vi "14-type_window.vi"(3 "this":i32, 4 "window in":i32, 5 "button":i32, 6 "settings in":T1={"Auto1"=TRUE, "Auto2"=TRUE, "Rel1"=TRUE, "Rel2"=TRUE, "Filt1"=TRUE, "Filt2"=TRUE, "Rate"=enum."Slow", "Range1"=enum."10mV", "Range2"=enum."100mV", "Filt3"=TRUE, "Filt4"=TRUE, "Rel temp 1"=TRUE, "Analog1"=FALSE, "Analog2"=FALSE, "Analog temp 1"=FALSE, "Digital1"=TRUE, "Digital2"=TRUE, "Digital temp 1 "=TRUE, "Window1"=enum."0,01%", "Window2"=enum."0,01%", "Window temp 1"=enum."0,01%", "RDGS1"="010", "RDGS2"="010", "RDGS temp 1"="010", "Type_type1"=TRUE, "Type_type2"=TRUE, "Type_type temp 1"=TRUE, "LSync"=FALSE, "Unit"=enum."C", "Sens"=TRUE, "Type tcoupl"=enum."J", "Junc"=TRUE, "prevState"=0, "Rel temp 2"=TRUE, "Analog temp 2"=FALSE, "Digital temp 2"=TRUE, "Type_type temp 2"=TRUE, "RDGS temp 2"="010", "Window temp 2"=enum."0,01%", "addres"=0}) -> (0 "next state":i32, 1 "window out":i32, 2 "settings out":T1)   [LabVIEW 2017]
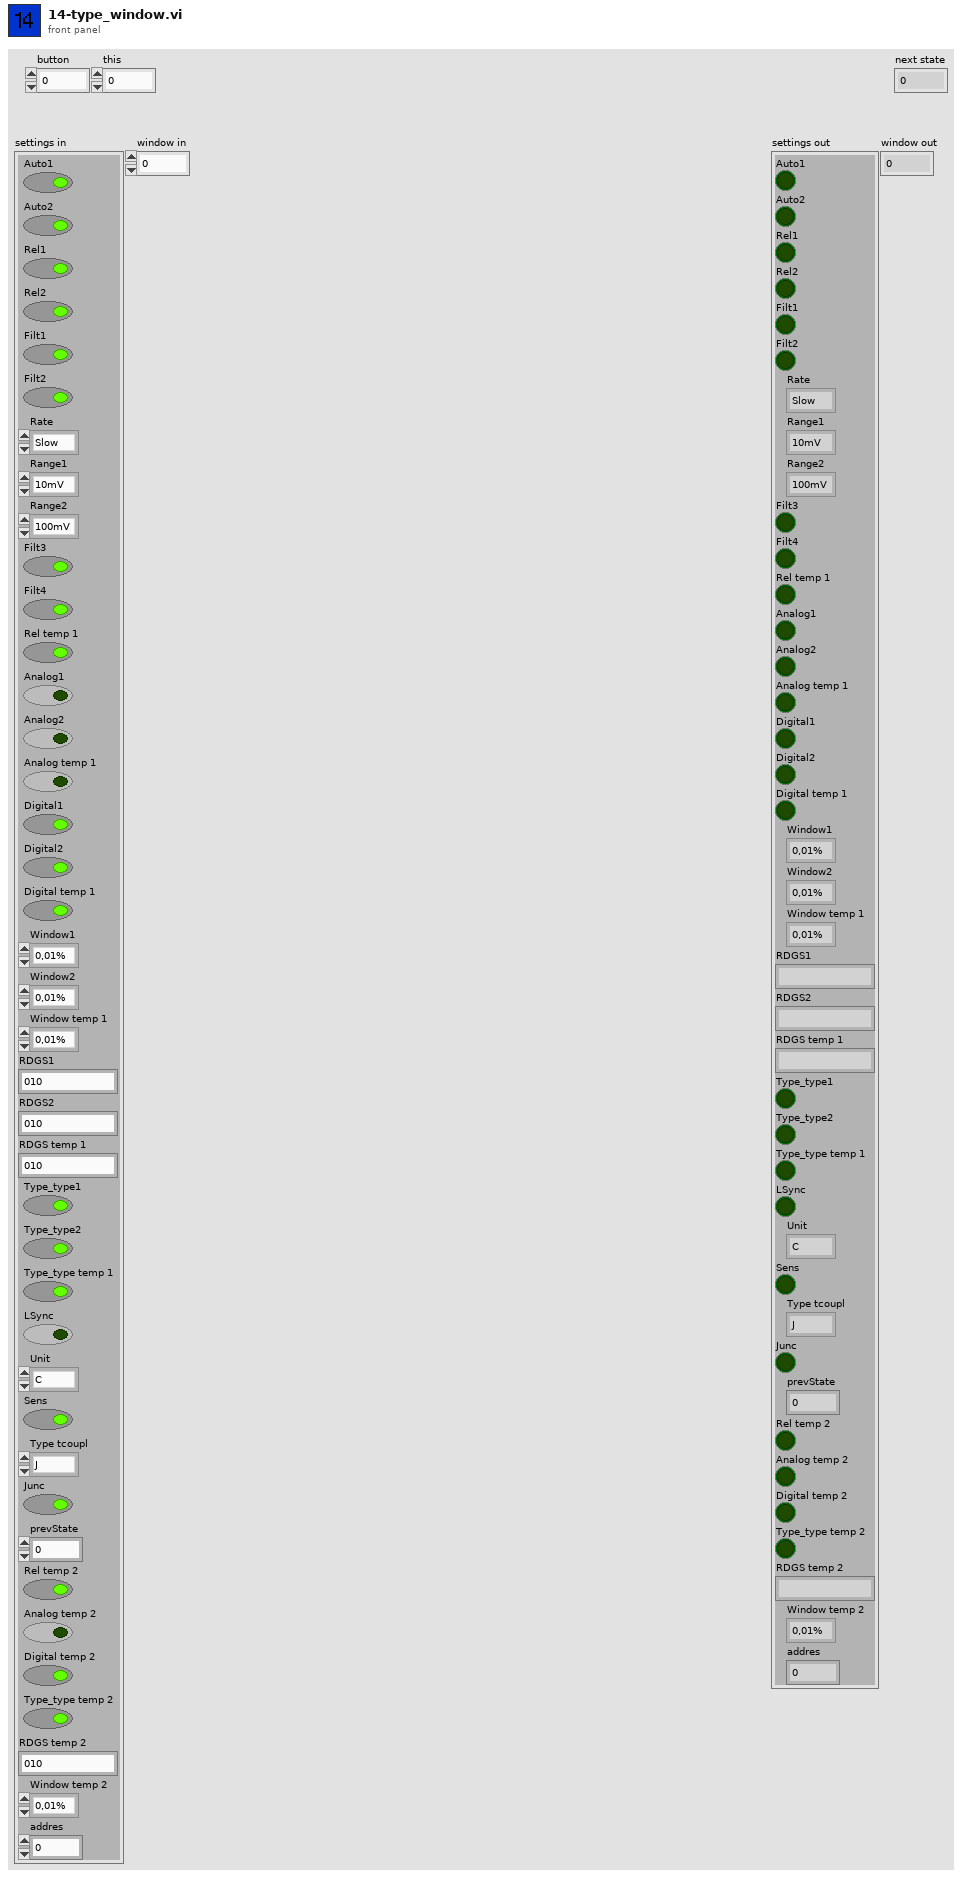
[diagram p1: front panel]
types:
  T1 = cluster{"Auto1":bool, "Auto2":bool, "Rel1":bool, "Rel2":bool, "Filt1":bool, "Filt2":bool, "Rate":enum16{"Slow", "Med", "Fast"}, "Range1":enum16{"10mV", "100mV", "1V", "10V", "100V"}, "Range2":enum16{"100mV", "1V", "10V"}, "Filt3":bool, "Filt4":bool, "Rel temp 1":bool, "Analog1":bool, "Analog2":bool, "Analog temp 1":bool, "Digital1":bool, "Digital2":bool, "Digital temp 1 ":bool, "Window1":enum16{"0,01%", "0,1%", "1%", "10%", "None"}, "Window2":enum16{"0,01%", "0,1%", "1%", "10%", "None"}, "Window temp 1":enum16{"0,01%", "0,1%", "1%", "10%", "None"}, "RDGS1":string, "RDGS2":string, "RDGS temp 1":string, "Type_type1":bool, "Type_type2":bool, "Type_type temp 1":bool, "LSync":bool, "Unit":enum16{"C", "K", "F"}, "Sens":bool, "Type tcoupl":enum16{"J", "K", "T", "E", "R", "S", "B", "N"}, "Junc":bool, "prevState":i32, "Rel temp 2":bool, "Analog temp 2":bool, "Digital temp 2":bool, "Type_type temp 2":bool, "RDGS temp 2":string, "Window temp 2":enum16{"0,01%", "0,1%", "1%", "10%", "None"}, "addres":i32}
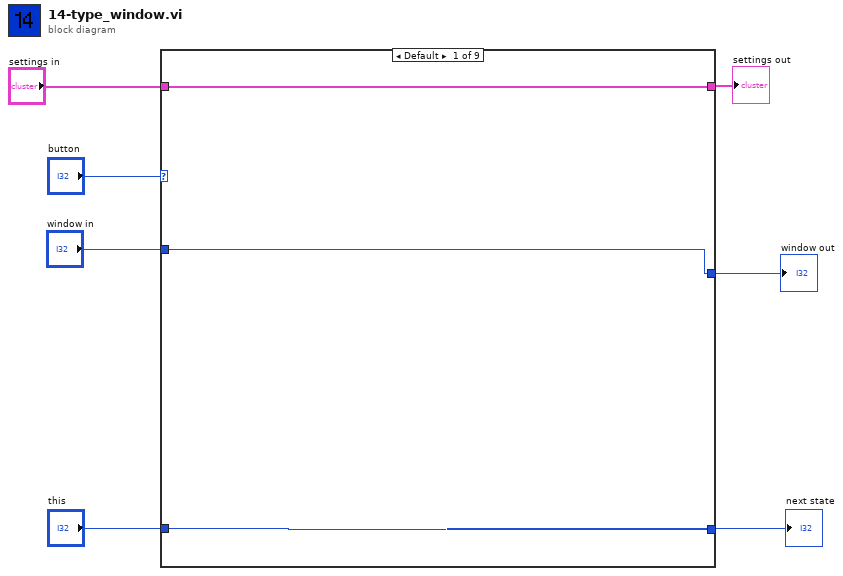
[diagram p0: block diagram]
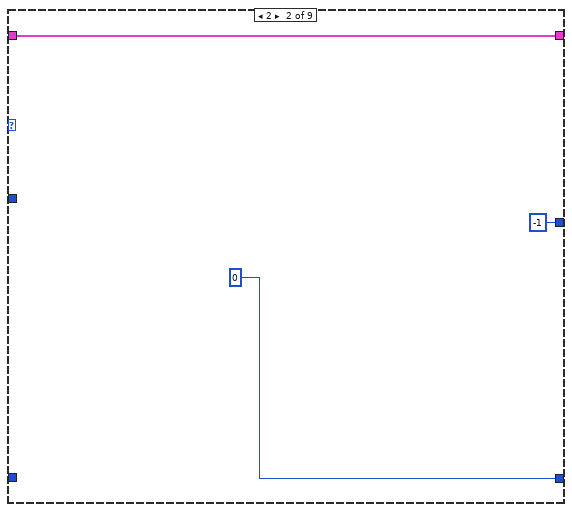
[diagram p2: hidden frame]
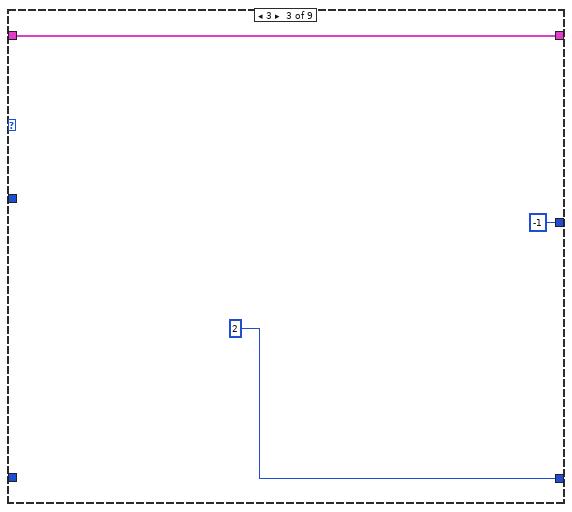
[diagram p3: hidden frame]
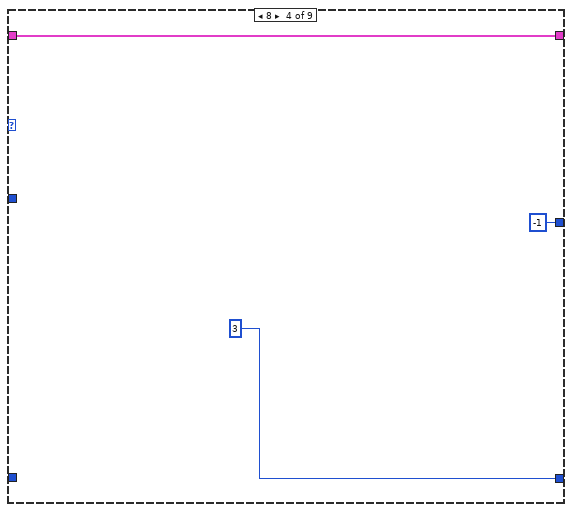
[diagram p4: hidden frame]
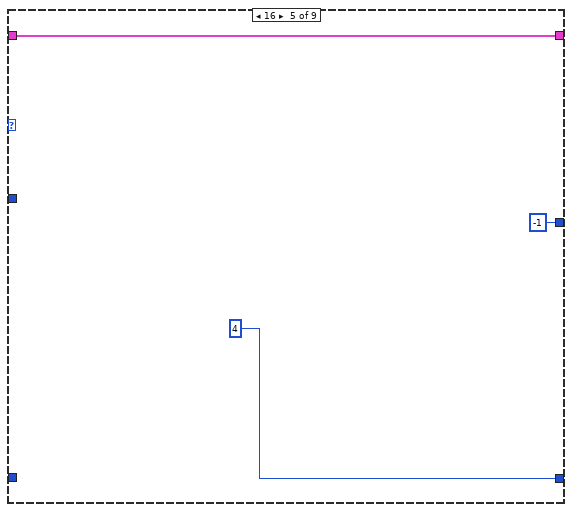
[diagram p5: hidden frame]
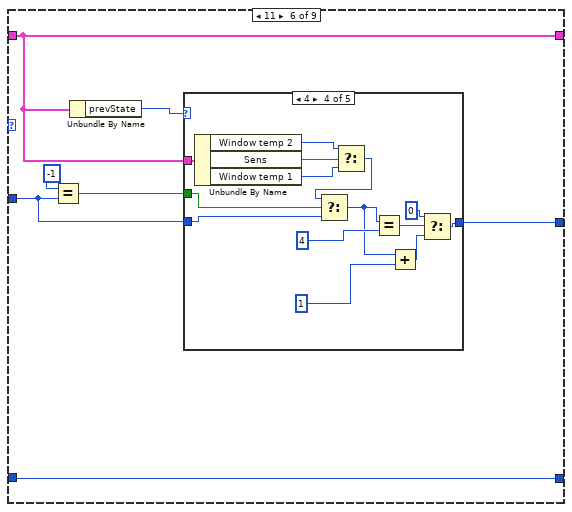
[diagram p6: hidden frame]
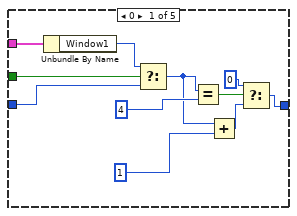
[diagram p7: hidden frame]
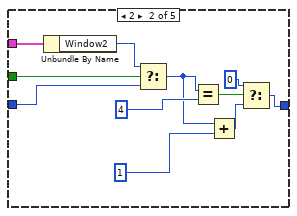
[diagram p8: hidden frame]
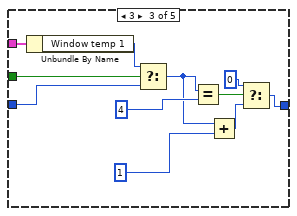
[diagram p9: hidden frame]
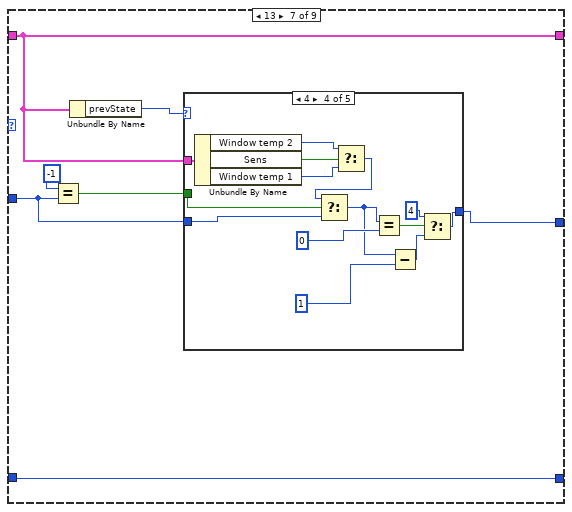
[diagram p11: hidden frame]
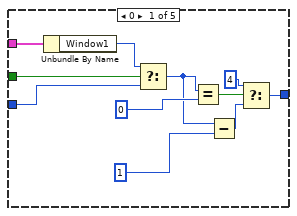
[diagram p12: hidden frame]
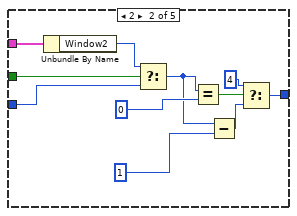
[diagram p13: hidden frame]
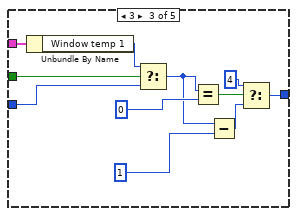
[diagram p14: hidden frame]
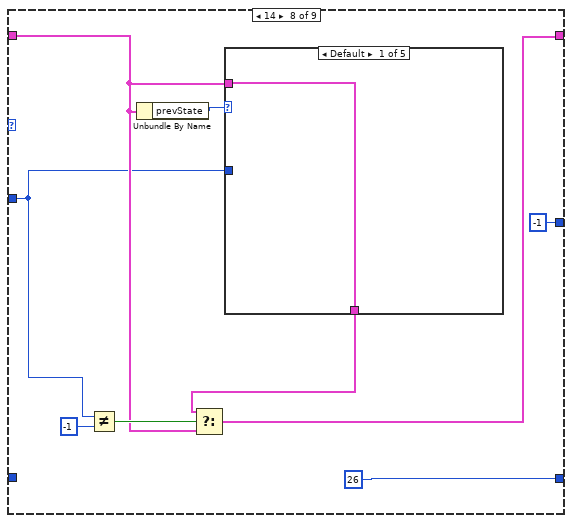
[diagram p16: hidden frame]
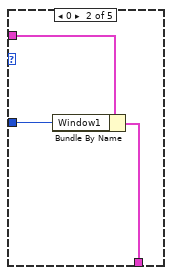
[diagram p17: hidden frame]
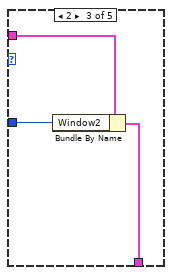
[diagram p18: hidden frame]
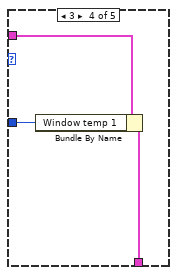
[diagram p19: hidden frame]
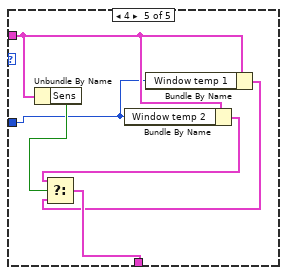
[diagram p20: hidden frame]
diagram:
  n1 = case shown="Default" "button" {
    tunnel: [w9 0 ("this") 2 3 4 w29 w84 26 ("this") w159] -> w5
    tunnel: "this" -> [w9 _ _ _ _ w29 w84 _ _]
    tunnel: "settings in" -> [w10 w13 w15 w18 w21 w25 w80 w137 w160]
    tunnel: [w10 w13 w15 w18 w21 w25 w80 w134 w160] -> w3
    tunnel: "window in" -> [w8 _ _ _ _ w26 w81 w136 _]
    tunnel: [w8 -1 ("window in") -1 ("window in") -1 ("window in") -1 ("window in") w23 w78 -1 ("window in") -1 ("window in")] -> w1
    frame Default {
    }
    frame 2 {
    }
    frame 3 {
    }
    frame 8 {
    }
    frame 16 {
    }
    frame 11 {
      n2 = Equal?(x=-1, y=w26) -> (x = y?=w27:bool)
      n3 = Unbundle By Name(w25) -> ("prevState"=w28:i32)
      n4 = case shown="4" w28 {
        tunnel: w27 -> [w35 w46 w57 w71 _]
        tunnel: w26 -> [w30 w41 w52 w68 w77]
        tunnel: w25 -> [w34 w45 w56 w67 _]
        tunnel: [w31 w42 w53 w69 w77] -> w23
        frame 0 {
          n5 = Unbundle By Name(w34) -> ("Window1"=w33:enum16{"0,01%", "0,1%", "1%", "10%", "None"})
          n6 = Select(t=w33, s=w35, f=w30) -> (s? t:f=w32:i32)
          n7 = Equal?(x=w32, y=4) -> (x = y?=w39:bool)
          n8 = Add(x=w32, y=1) -> (x+y=w40:i32)
          n9 = Select(t=0, s=w39, f=w40) -> (s? t:f=w31:i32)
        }
        frame 2 {
          n10 = Unbundle By Name(w45) -> ("Window2"=w44:enum16{"0,01%", "0,1%", "1%", "10%", "None"})
          n11 = Select(t=w44, s=w46, f=w41) -> (s? t:f=w43:i32)
          n12 = Equal?(x=w43, y=4) -> (x = y?=w50:bool)
          n13 = Add(x=w43, y=1) -> (x+y=w51:i32)
          n14 = Select(t=0, s=w50, f=w51) -> (s? t:f=w42:i32)
        }
        frame 3 {
          n15 = Unbundle By Name(w56) -> ("Window temp 1"=w55:enum16{"0,01%", "0,1%", "1%", "10%", "None"})
          n16 = Select(t=w55, s=w57, f=w52) -> (s? t:f=w54:i32)
          n17 = Equal?(x=w54, y=4) -> (x = y?=w61:bool)
          n18 = Add(x=w54, y=1) -> (x+y=w62:i32)
          n19 = Select(t=0, s=w61, f=w62) -> (s? t:f=w53:i32)
        }
        frame 4 {
          n20 = Unbundle By Name(w67) -> ("Window temp 2"=w65:enum16{"0,01%", "0,1%", "1%", "10%", "None"}, "Sens"=w66:bool, "Window temp 1"=w64:enum16{"0,01%", "0,1%", "1%", "10%", "None"})
          n21 = Select(t=w65, s=w66, f=w64) -> (s? t:f=w63:enum16{"0,01%", "0,1%", "1%", "10%", "None"})
          n22 = Select(t=w63, s=w71, f=w68) -> (s? t:f=w70:i32)
          n23 = Equal?(x=w70, y=4) -> (x = y?=w75:bool)
          n24 = Add(x=w70, y=1) -> (x+y=w76:i32)
          n25 = Select(t=0, s=w75, f=w76) -> (s? t:f=w69:i32)
        }
        frame Default {
        }
      }
    }
    frame 13 {
      n26 = Equal?(x=-1, y=w81) -> (x = y?=w82:bool)
      n27 = Unbundle By Name(w80) -> ("prevState"=w83:i32)
      n28 = case shown="4" w83 {
        tunnel: w82 -> [w90 w101 w112 w126 _]
        tunnel: w81 -> [w85 w96 w107 w123 w132]
        tunnel: w80 -> [w89 w100 w111 w122 _]
        tunnel: [w86 w97 w108 w124 w132] -> w78
        frame 0 {
          n29 = Unbundle By Name(w89) -> ("Window1"=w88:enum16{"0,01%", "0,1%", "1%", "10%", "None"})
          n30 = Select(t=w88, s=w90, f=w85) -> (s? t:f=w87:i32)
          n31 = Equal?(x=w87, y=0) -> (x = y?=w94:bool)
          n32 = Subtract(x=w87, y=1) -> (x-y=w95:i32)
          n33 = Select(t=4, s=w94, f=w95) -> (s? t:f=w86:i32)
        }
        frame 2 {
          n34 = Unbundle By Name(w100) -> ("Window2"=w99:enum16{"0,01%", "0,1%", "1%", "10%", "None"})
          n35 = Select(t=w99, s=w101, f=w96) -> (s? t:f=w98:i32)
          n36 = Equal?(x=w98, y=0) -> (x = y?=w105:bool)
          n37 = Subtract(x=w98, y=1) -> (x-y=w106:i32)
          n38 = Select(t=4, s=w105, f=w106) -> (s? t:f=w97:i32)
        }
        frame 3 {
          n39 = Unbundle By Name(w111) -> ("Window temp 1"=w110:enum16{"0,01%", "0,1%", "1%", "10%", "None"})
          n40 = Select(t=w110, s=w112, f=w107) -> (s? t:f=w109:i32)
          n41 = Equal?(x=w109, y=0) -> (x = y?=w116:bool)
          n42 = Subtract(x=w109, y=1) -> (x-y=w117:i32)
          n43 = Select(t=4, s=w116, f=w117) -> (s? t:f=w108:i32)
        }
        frame 4 {
          n44 = Unbundle By Name(w122) -> ("Window temp 2"=w120:enum16{"0,01%", "0,1%", "1%", "10%", "None"}, "Sens"=w121:bool, "Window temp 1"=w119:enum16{"0,01%", "0,1%", "1%", "10%", "None"})
          n45 = Select(t=w120, s=w121, f=w119) -> (s? t:f=w118:enum16{"0,01%", "0,1%", "1%", "10%", "None"})
          n46 = Select(t=w118, s=w126, f=w123) -> (s? t:f=w125:i32)
          n47 = Equal?(x=w125, y=0) -> (x = y?=w130:bool)
          n48 = Subtract(x=w125, y=1) -> (x-y=w131:i32)
          n49 = Select(t=4, s=w130, f=w131) -> (s? t:f=w124:i32)
        }
        frame Default {
        }
      }
    }
    frame 14 {
      n50 = Not Equal?(x=w136, y=-1) -> (x != y?=w139:bool)
      n51 = Unbundle By Name(w137) -> ("prevState"=w138:i32)
      n52 = case shown="Default" w138 {
        tunnel: w137 -> [w142 w145 w148 w151 w157]
        tunnel: w136 -> [_ w144 w147 w150 w153]
        tunnel: [w142 w143 w146 w149 w156] -> w135
        frame Default {
        }
        frame 0 {
          n53 = Bundle By Name(cluster=w145, "Window1"=w144) -> (w143:T1)
        }
        frame 2 {
          n54 = Bundle By Name(cluster=w148, "Window2"=w147) -> (w146:T1)
        }
        frame 3 {
          n55 = Bundle By Name(cluster=w151, "Window temp 1"=w150) -> (w149:T1)
        }
        frame 4 {
          n56 = Unbundle By Name(w157) -> ("Sens"=w155:bool)
          n57 = Bundle By Name(cluster=w157, "Window temp 2"=w153) -> (w154:T1)
          n58 = Bundle By Name(cluster=w157, "Window temp 1"=w153) -> (w152:T1)
          n59 = Select(t=w154, s=w155, f=w152) -> (s? t:f=w156:T1)
        }
      }
      n60 = Select(t=w135, s=w139, f=w137) -> (s? t:f=w134:T1)
    }
    frame 32 {
      n61 = Unbundle By Name(w160) -> ("prevState"=w159:i32)
    }
  }
  "next state" <- w5
  "settings out" <- w3
  "window out" <- w1
